vi "Target2.vi"   [LabVIEW 2025]
uses:
  <vilib>/eio/utilities/niEioResolveVilibRelativePath.vi
  <vilib>/rvi/interface/RandomDataEmulation/niFpgaRandomDataHandleErrors.vi
  <vilib>/rvi/Memory/Memory_Emulation/nirvimemoryFastEmulation.vi
  <vilib>/rvi/Memory/Memory_Emulation/nirvimemoryEmulation.vi
  <vilib>/rvi/Emulation/niFpgaEmulationIsFPGAContextNoSignature.vi
  <vilib>/rvi/DataTransferAndStorage/Container/Common/niFpgaContainerGetUniqueNameForEmu.vi
  <vilib>/rvi/Emulation/niFpgaProcessEmulError.vi
  <vilib>/rvi/Emulation/niFpgaSctlEmulationGetInTimedLoop.vi
  <vilib>/rvi/errors/nirviReportUnexpectedCaseInternalError (U32).vi
  <vilib>/ARTS-Lab/Array-based Linear Algebra/vector_matrix_multiply_VIs/vector_matrix_multiply_SGL.vi
  <vilib>/ARTS-Lab/Array-based Linear Algebra/matrix_matrix_VIs/matrix_matrix_multiply_SGL.vi
  <vilib>/rvi/DataTransferAndStorage/Container/XNode/niFpgaContainer.xnode
  <vilib>/rvi/interface/RandomDataEmulation/nirviRandomDataFpgaReadWriteTemplate.vi
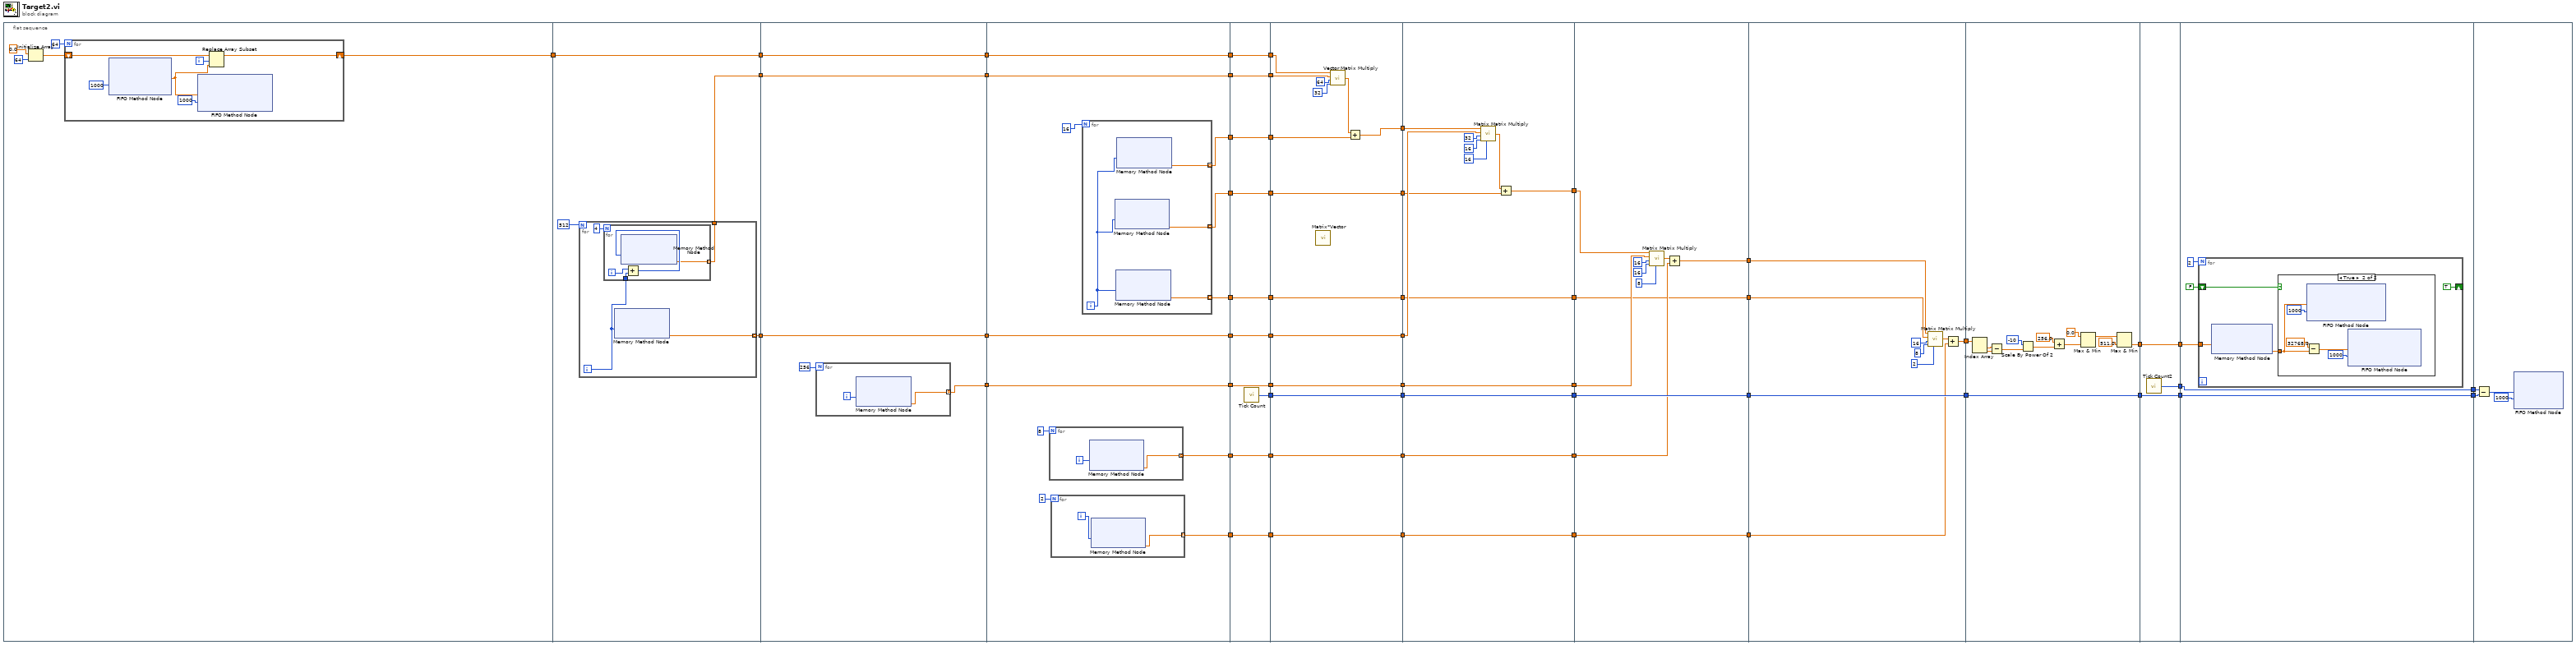
[diagram p0: block diagram]
diagram:
  n1 = flat-sequence {
    tunnel: [w58] -> w35
    tunnel: w35 -> [w69]
    tunnel: [w69] -> w34
    tunnel: [w67] -> w29
    tunnel: [w66] -> w25
    tunnel: w34 -> [w82]
    tunnel: [w82] -> w36
    tunnel: [w80] -> w30
    tunnel: w29 -> [w80]
    tunnel: [w79] -> w26
    tunnel: w25 -> [w79]
    tunnel: [w78] -> w15
    tunnel: w36 -> [w96]
    tunnel: [w96] -> w37
    tunnel: [w92] -> w31
    tunnel: w30 -> [w92]
    tunnel: [w91] -> w27
    tunnel: w26 -> [w91]
    tunnel: [w90] -> w23
    tunnel: [w89] -> w20
    tunnel: [w88] -> w16
    tunnel: w15 -> [w88]
    tunnel: [w87] -> w14
    tunnel: [w86] -> w6
    tunnel: [w85] -> w1
    tunnel: w37 -> [w114]
    tunnel: [w114] -> w44
    tunnel: [w113] -> w45
    tunnel: [w112] -> w32
    tunnel: w31 -> [w112]
    tunnel: [w111] -> w28
    tunnel: w27 -> [w111]
    tunnel: [w110] -> w24
    tunnel: w23 -> [w110]
    tunnel: [w109] -> w21
    tunnel: w20 -> [w109]
    tunnel: [w108] -> w17
    tunnel: w16 -> [w108]
    tunnel: w14 -> [w107]
    tunnel: [w107] -> w13
    tunnel: [w106] -> w7
    tunnel: w6 -> [w106]
    tunnel: [w105] -> w2
    tunnel: w1 -> [w105]
    tunnel: w45 -> [w128]
    tunnel: [w128] -> w43
    tunnel: w44 -> [w123]
    tunnel: [w124] -> w42
    tunnel: [w122] -> w33
    tunnel: w32 -> [w122]
    tunnel: w28 -> [w121]
    tunnel: w24 -> [w120]
    tunnel: [w119] -> w22
    tunnel: w21 -> [w119]
    tunnel: [w118] -> w18
    tunnel: w17 -> [w118]
    tunnel: w13 -> [w117]
    tunnel: [w117] -> w12
    tunnel: [w116] -> w8
    tunnel: w7 -> [w116]
    tunnel: [w115] -> w3
    tunnel: w2 -> [w115]
    tunnel: w43 -> [w141]
    tunnel: [w141] -> w41
    tunnel: w42 -> [w135]
    tunnel: [w136] -> w39
    tunnel: w33 -> [w134]
    tunnel: w22 -> [w133]
    tunnel: [w132] -> w19
    tunnel: w18 -> [w132]
    tunnel: w12 -> [w131]
    tunnel: [w131] -> w11
    tunnel: [w130] -> w9
    tunnel: w8 -> [w130]
    tunnel: [w129] -> w4
    tunnel: w3 -> [w129]
    tunnel: w41 -> [w152]
    tunnel: [w152] -> w40
    tunnel: w39 -> [w146]
    tunnel: [w147] -> w38
    tunnel: w19 -> [w145]
    tunnel: w11 -> [w144]
    tunnel: [w143] -> w10
    tunnel: w9 -> [w143]
    tunnel: [w142] -> w5
    tunnel: w4 -> [w142]
    tunnel: [w156] -> w54
    tunnel: [w161] -> w53
    tunnel: w40 -> [w161]
    tunnel: w38 -> [w155]
    tunnel: w10 -> [w154]
    tunnel: w5 -> [w153]
    tunnel: w54 -> [w164]
    tunnel: [w163] -> w52
    tunnel: w53 -> [w162]
    tunnel: [w162] -> w51
    tunnel: w52 -> [w177]
    tunnel: [w177] -> w50
    tunnel: w51 -> [w176]
    tunnel: [w176] -> w49
    tunnel: [w175] -> w48
    tunnel: w50 -> [w181]
    tunnel: [w178] -> w47
    tunnel: w49 -> [w179]
    tunnel: [w179] -> w46
    tunnel: w48 -> [w178]
    tunnel: w47 -> [w195]
    tunnel: w46 -> [w194]
    frame #0 {
      n2 = Initialize Array(sgl 0.0 ("element"), 64 ("dimension size")) -> (w55:sgl[])
      n3 = for {
        N: 64 -> [_]
        shift-right: [w61] -> w58
        shift-left: w55 -> [w63]
        i -> [w60]
        n4 = xnode ("FIFO Method Node")("Timeout"=1000) -> ("Element"=w62:sgl)  [unwired: 1 in, 2 out]
        n5 = xnode ("FIFO Method Node")("Element"=w62, "Timeout"=1000) -> ()  [unwired: 1 in, 2 out]
        n6 = Replace Array Subset(array=w63, new element=w62, index=w60) -> (w61:sgl[])
      }
    }
    frame #1 {
      n7 = for {
        N: 512 -> [_]
        tunnel: [w71] -> w67 mode=indexing
        tunnel: [w70] -> w66
        i -> [w72]
        n8 = for {
          N: 4 -> [_]
          tunnel: w72 -> [w76]
          tunnel: [w74] -> w70 mode=indexing
          i -> [w77]
          n9 = Add(x=w77, y=w76) -> (x+y=w75:i32)
          n10 = xnode ("Memory Method Node")("Address"=w75) -> ("Data"=w74:sgl)  [unwired: 1 in, 1 out]
        }
        n11 = xnode ("Memory Method Node")("Address"=w72) -> ("Data"=w71:sgl)  [unwired: 1 in, 1 out]
      }
    }
    frame #2 {
      n12 = for {
        N: 256 -> [_]
        tunnel: [w83] -> w78 mode=indexing
        i -> [w84]
        n13 = xnode ("Memory Method Node")("Address"=w84) -> ("Data"=w83:sgl)  [unwired: 1 in, 1 out]
      }
    }
    frame #3 {
      n14 = for {
        N: 8 -> [_]
        tunnel: [w99] -> w87 mode=indexing
        i -> [w100]
        n15 = xnode ("Memory Method Node")("Address"=w100) -> ("Data"=w99:sgl)  [unwired: 1 in, 1 out]
      }
      n16 = for {
        N: 2 -> [_]
        tunnel: [w97] -> w86 mode=indexing
        i -> [w98]
        n17 = xnode ("Memory Method Node")("Address"=w98) -> ("Data"=w97:sgl)  [unwired: 1 in, 1 out]
      }
      n18 = for {
        N: 16 -> [_]
        tunnel: [w103] -> w90 mode=indexing
        tunnel: [w102] -> w89 mode=indexing
        tunnel: [w101] -> w85 mode=indexing
        i -> [w104]
        n19 = xnode ("Memory Method Node")("Address"=w104) -> ("Data"=w102:sgl)  [unwired: 1 in, 1 out]
        n20 = xnode ("Memory Method Node")("Address"=w104) -> ("Data"=w101:sgl)  [unwired: 1 in, 1 out]
        n21 = xnode ("Memory Method Node")("Address"=w104) -> ("Data"=w103:sgl)  [unwired: 1 in, 1 out]
      }
    }
    frame #4 {
      n22 = call "Tick Count"() -> ("Tick Count(uSec)"=w113:u32)
    }
    frame #5 {
      n23 = call "Matrix*Vector"() -> ()  [unwired: 11 in, 1 out]
      n24 = call-poly <vilib>:"Vector Matrix Multiply.vi"("p"=32, "n"=64, "B"=w121, "A"=w123) -> ("C"=w127:sgl[])
      n25 = Add(x=w127, y=w120) -> (x+y=w124:sgl[])
    }
    frame #6 {
      n26 = call-poly <vilib>:"Matrix Matrix Multiply.vi"("p"=16 ("n"), "n"=16, "m"=32, "B"=w134, "A"=w135) -> ("C"=w140:sgl[])  [unwired: 1 in]
      n27 = Add(x=w140, y=w133) -> (x+y=w136:sgl[])
    }
    frame #7 {
      n28 = call-poly <vilib>:"Matrix Matrix Multiply.vi"("p"=8, "n"=16, "m"=16, "B"=w145, "A"=w146) -> ("C"=w151:sgl[])  [unwired: 1 in]
      n29 = Add(x=w151, y=w144) -> (x+y=w147:sgl[])
    }
    frame #8 {
      n30 = call-poly <vilib>:"Matrix Matrix Multiply.vi"("p"=2, "n"=8, "m"=16, "B"=w153, "A"=w155) -> ("C"=w158:sgl[])  [unwired: 1 in]
      n31 = Add(x=w158, y=w154) -> (x+y=w156:sgl[])
    }
    frame #9 {
      n32 = Index Array(array=w164) -> (element #1=w169:sgl, element #2=w170:sgl)  [unwired: 2 in]
      n33 = Subtract(x=w169, y=w170) -> (x-y=w171:sgl)
      n34 = Scale By Power Of 2(n=i16 -10, x=w171) -> (x*2^n=w172:sgl)
      n35 = Add(x=sgl 256.0, y=w172) -> (x+y=w173:sgl)
      n36 = Max & Min(x=sgl 0.0, y=w173) -> (max(x,y)=w174:sgl)  [unwired: 1 out]
      n37 = Max & Min(x=w174, y=sgl 511.0) -> (min(x,y)=w163:sgl)  [unwired: 1 out]
    }
    frame #10 {
      n38 = call "Tick Count2"() -> ("Tick Count(uSec)"=w175:u32)
    }
    frame #11 {
      n39 = for {
        N: 2 -> [_]
        tunnel: w181 -> [w186]
        shift-right: [TRUE] -> _
        shift-left: FALSE -> [w185]
        n40 = xnode ("Memory Method Node")("Address"=w186) -> ("Data"=w183:sgl)  [unwired: 1 in, 1 out]
        n41 = case shown="True" w185 {
          tunnel: w183 -> [_ w187]
          frame False {
          }
          frame True {
            n42 = xnode ("FIFO Method Node")("Element"=w187, "Timeout"=1000) -> ()  [unwired: 1 in, 2 out]
            n43 = Subtract(x=sgl 32768.0, y=w187) -> (x-y=w191:sgl)
            n44 = xnode ("FIFO Method Node")("Element"=w191, "Timeout"=1000) -> ()  [unwired: 1 in, 2 out]
          }
        }
      }
    }
    frame #12 {
      n45 = Subtract(x=w195, y=w194) -> (x-y=w193:u32)
      n46 = xnode ("FIFO Method Node")("Element"=w193, "Timeout"=1000) -> ()  [unwired: 1 in, 2 out]
    }
  }
